vi "LeastDistanceAngle.vi"(3 "Enum":enum16{"within pi", "within pi/2"}(ring)=enum."within pi/2", 4 "Current angle":dbl, 5 "target angle (between pi and -pi) 2":dbl(knob) scale=3.14159..-3.14159) -> (0 "current angle (between pi and -pi) 2":dbl(knob) scale=3.14159..-3.14159, 1 "Reverse?":bool, 2 "output angle":dbl)   [LabVIEW 2014, in "Team900SwerveDrive.lvlib"]
uses:
  Team900SwerveDrive.lvlib
panel:
  out "within pi":dbl(knob) scale=3.14159..-3.14159
  out "within pi/2":dbl(knob) scale=3.14159..-3.14159
  out "straightforward delta":dbl(knob) scale=3.14159..-3.14159
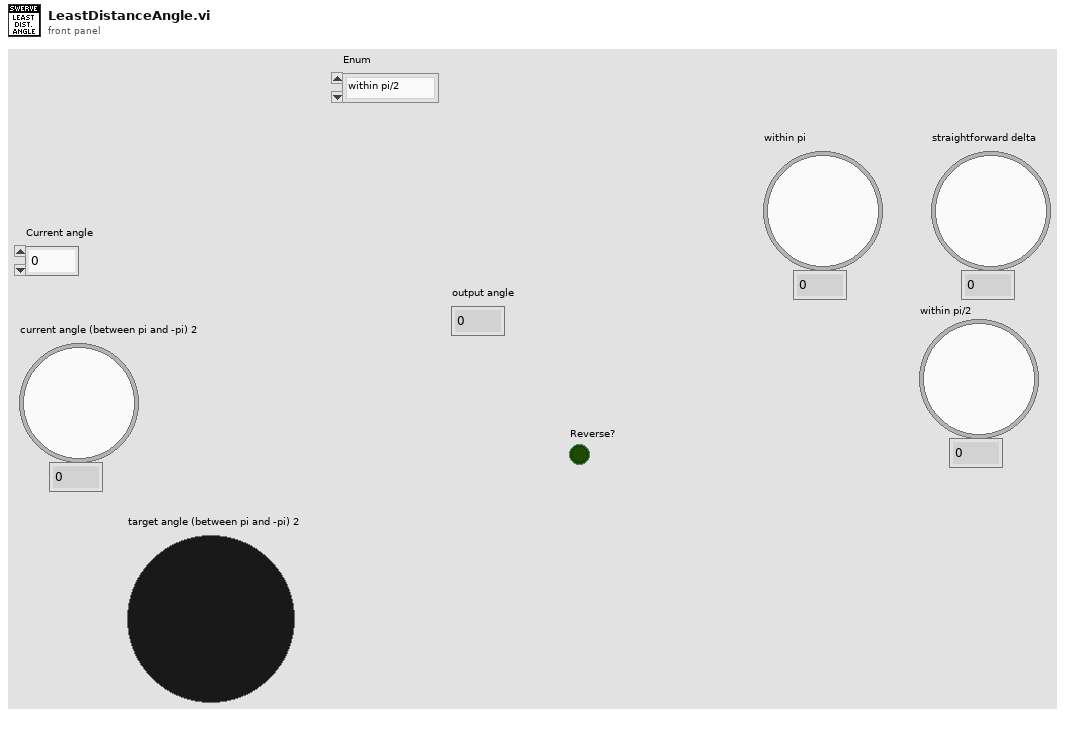
[diagram p1: front panel]
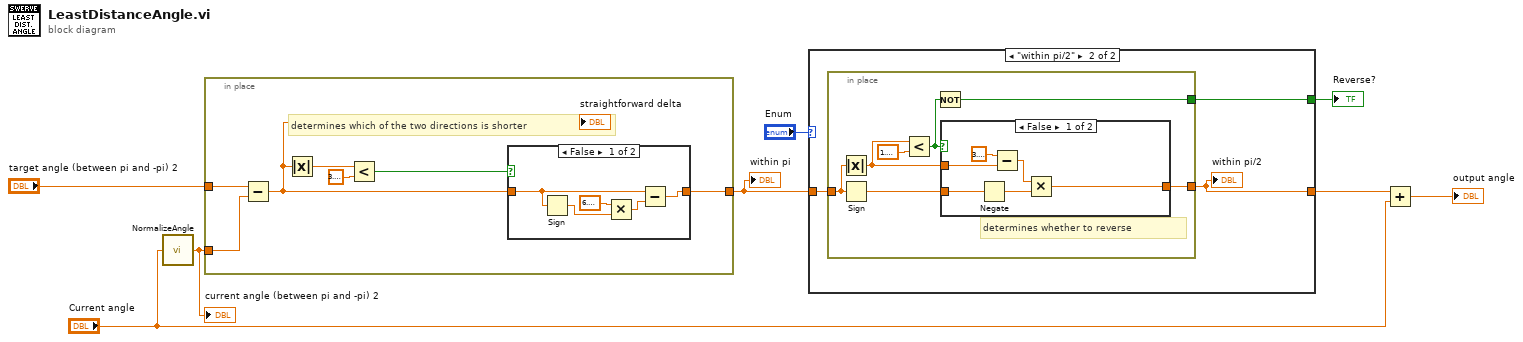
[diagram p0: block diagram]
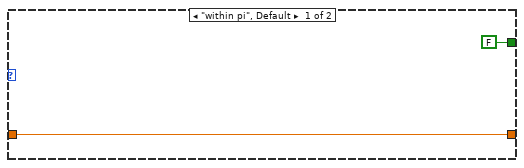
[diagram p2: hidden frame]
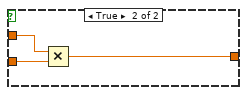
[diagram p3: hidden frame]
diagram:
  n1 = call "NormalizeAngle.vi"("angle (rad)"="Current angle") -> ("angle (between pi and -pi)"=w7:dbl)
  "current angle (between pi and -pi) 2" <- w7
  n2 = in-place {
    in-place-border: "target angle (between pi and -pi) 2" -> [w10]
    in-place-border: w7 -> [w9]
    in-place-border: [w11] -> w8
    # "determines which of the two directions is shorter"
    n3 = Subtract(x=w10, y=w9) -> (x-y=w15:dbl)
    "straightforward delta" <- w15
    n4 = Absolute Value(x=w15) -> (abs(x)=w14:dbl)
    n5 = Less?(x=w14, y=3.141592653589793) -> (x < y?=w13:bool)
    n6 = case shown="False" w13 {
      tunnel: w15 -> [w17 w21]
      tunnel: [w16 w21] -> w11
      frame False {
        n7 = Sign(1:w17) -> (0:w19:dbl)
        n8 = Multiply(x=6.283185307179586, y=w19) -> (x*y=w18:dbl)
        n9 = Subtract(x=w17, y=w18) -> (x-y=w16:dbl)
      }
      frame True {
      }
    }
  }
  "within pi" <- w8
  n10 = case shown="\"within pi/2\"" "Enum" {
    tunnel: w8 -> [w23 w26]
    tunnel: [w23 w24] -> w6
    tunnel: [FALSE w25] -> w3
    frame "within pi", Default {
    }
    frame "within pi/2" {
      n11 = in-place {
        in-place-border: w26 -> [w33]
        in-place-border: [w29] -> w24
        in-place-border: [w27] -> w25
        # "determines whether to reverse"
        n12 = Absolute Value(x=w33) -> (abs(x)=w30:dbl)
        n13 = Sign(1:w33) -> (0:w31:dbl)
        n14 = Less?(x=w30, y=1.5707963267948966) -> (x < y?=w28:bool)
        n15 = Not(x=w28) -> (.not. x?=w27:bool)
        n16 = case shown="False" w28 {
          tunnel: w31 -> [w36 w41]
          tunnel: w30 -> [w39 w42]
          tunnel: [w35 w40] -> w29
          frame False {
            n17 = Negate(x=w36) -> (-x=w34:dbl)
            n18 = Subtract(x=3.141592653589793, y=w39) -> (x-y=w37:dbl)
            n19 = Multiply(x=w37, y=w34) -> (x*y=w35:dbl)
          }
          frame True {
            n20 = Multiply(x=w42, y=w41) -> (x*y=w40:dbl)
          }
        }
      }
      "within pi/2" <- w24
    }
  }
  "Reverse?" <- w3
  n21 = Add(x=w6, y="Current angle") -> (x+y=→"output angle":dbl)
